vi "FF_AnkleTrajAdv.vi"(6 "Init":bool, 7 "dt":dbl=0.01 format="%0.2f", 8 "error in (no error)":errorcluster, 9 "AnkleVelocity":dbl[](array[numeric]), 10 "AnkleInGCS":dbl[](array[numeric]), 11 "Force Field Controller in":refnum<class "ForceField.lvclass">) -> (0 "error out":errorcluster, 1 "ClosestPoint":dbl[](array[numeric]), 2 "ForceXYZ":dbl[](array[numeric]), 3 "Force Field Controller out":refnum<class "ForceField.lvclass">, 4 "UpdateTrajPrev":bool, 5 "ForceNTD":dbl[](array[numeric]))   [LabVIEW 2016, in "ForceField.lvclass"]
uses:
  ForceField.lvclass
  ForceField.lvclass/ForceField.ctl
  <vilib>/ptbypt/NI_PtbyPt.lvlib
panel:
  out "ToeOffIdx":i32
  in  "3D":bool
  in  "Adv?":bool=TRUE
  out "weightPrev":dbl
  out "ClosePt 2":dbl[](array[numeric])
  in  "HalfWindow 2":i32=35
  in  "dXmin":dbl=0.2 format="%#_13g"
  in  "HalfWindow 1":i32=35
  out "ClosePt 1":dbl[](array[numeric])
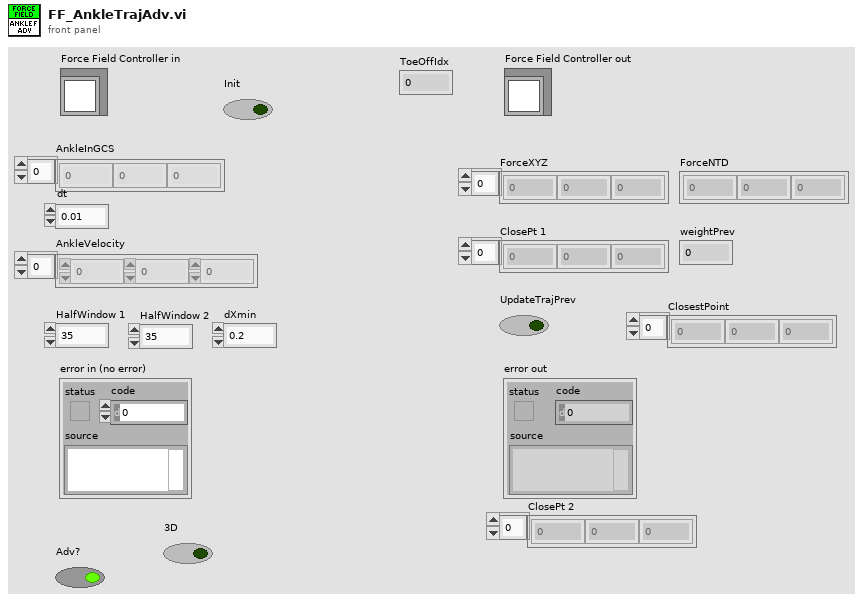
[diagram p1: front panel]
types:
  T1 = typedef "ForceField.lvclass/AnkleTrajPt.ctl" = cluster{"P1":dbl[], "P2":dbl[], "P1-P2":dbl[], "(P1-P2)^2":dbl}
  T2 = typedef "ForceField.lvclass/ForceNTD.ctl" = cluster{"Vn":dbl[], "Vt":dbl[], "Dmin":dbl}
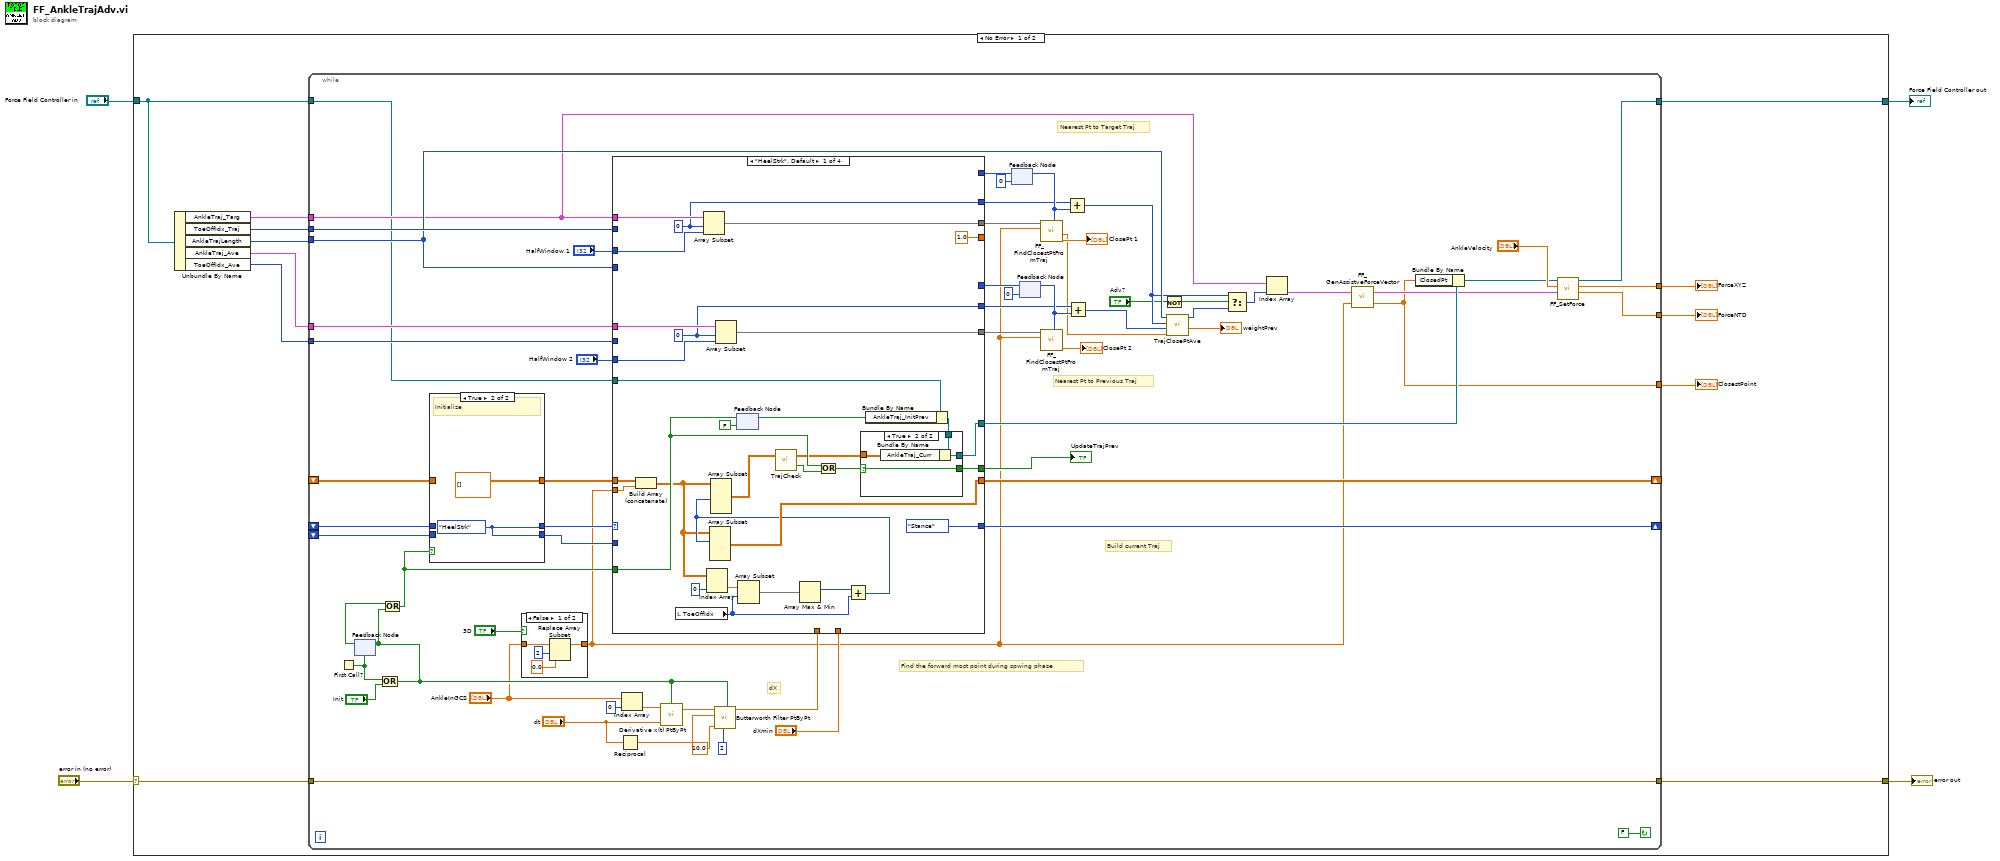
[diagram p0: block diagram]
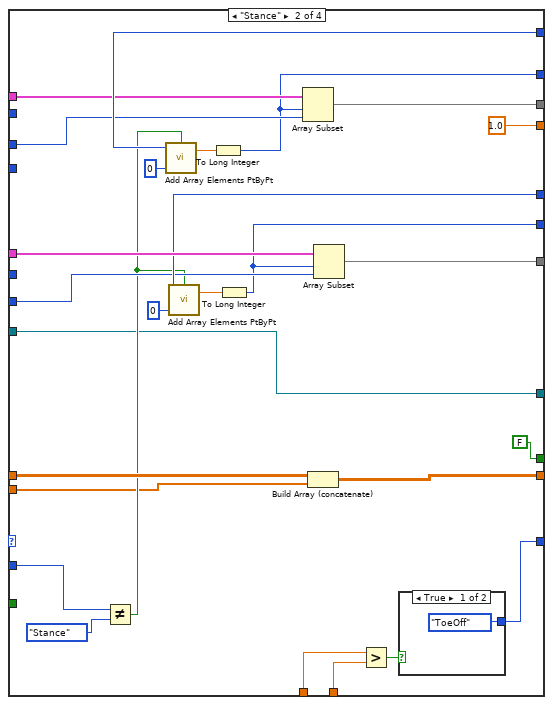
[diagram p4: hidden frame]
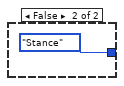
[diagram p5: hidden frame]
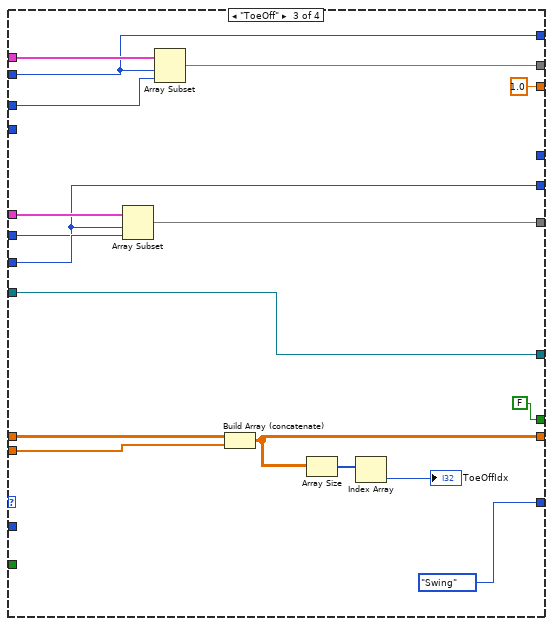
[diagram p6: hidden frame]
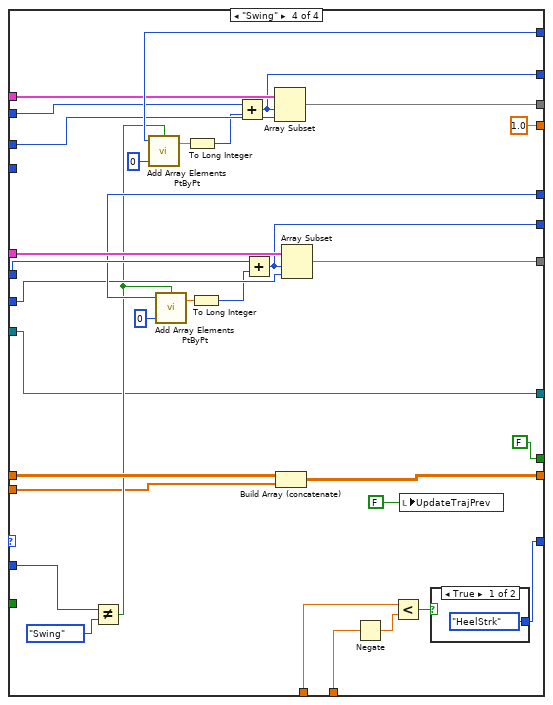
[diagram p7: hidden frame]
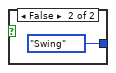
[diagram p8: hidden frame]
diagram:
  n1 = case shown="No Error" "error in (no error)" {
    selector: "error in (no error)" -> [w10 w211]
    tunnel: [w5 w211] -> w3
    tunnel: [w9 w210] -> w1
    tunnel: "Force Field Controller in" -> [w16 w210]
    frame No Error {
      n2 = Unbundle By Name(w16) -> ("AnkleTraj_Targ"=w15:T1[], "ToeOffIdx_Traj"=w14:i32, "AnkleTrajLength"=w13:i32, "AnkleTraj_Ave"=w12:T1[], "ToeOffIdx_Ave"=w11:i32)
      n3 = while {
        tunnel: w15 -> [w65]
        tunnel: w14 -> [w75]
        tunnel: w16 -> [w42]
        tunnel: [w21] -> w9
        shift-right: [w78] -> _
        shift-left: _ -> [w70]
        shift-left: _ -> [w68]
        shift-right: [w77] -> _
        shift-left: _ -> [w72]
        tunnel: w13 -> [w73]
        tunnel: w12 -> [w76]
        tunnel: w11 -> [w74]
        tunnel: w10 -> [w17]
        tunnel: [w20] -> w8
        tunnel: [w19] -> w7
        tunnel: [w18] -> w6
        tunnel: [w17] -> w5
        stop <- FALSE continue-if-true
        # "dX"
        # "Find the forward most point during spwing phase"
        # "Nearest Pt to Previous Traj"
        # "Build current Traj"
        # "Nearest Pt to Target Traj"
        n4 = First Call?() -> (First Call?: T/F=w28:bool)
        n5 = feedback #1(w28) -> (w66:bool)
        n6 = Or(x=w28, y="Init") -> (x .or. y?=w38:bool)
        n7 = feedback-in #1(w38) -> ()
        n8 = Or(x=w66, y=w38) -> (x .or. y?=w63:bool)
        n9 = case shown="True" w63 {
          tunnel: w72 -> [w207 _]
          tunnel: [w207 dbl[][] []] -> w71
          tunnel: w70 -> [w206 _]
          tunnel: [w206 w208] -> w69
          tunnel: w68 -> [w205 _]
          tunnel: [w205 w208] -> w67
          frame False {
          }
          frame True {
            w208 = enum16{"HeelStrk", "Stance", "ToeOff", "Swing"}."HeelStrk"
            # "Initialize"
          }
        }
        n10 = case shown="False" "3D" {
          tunnel: "AnkleInGCS" -> [w85 w86]
          tunnel: [w84 w86] -> w25
          frame False {
            n11 = Replace Array Subset(array=w85, new element=0.0 ("new element/subarray"), index=2) -> (w84:dbl[])
          }
          frame True {
          }
        }
        n12 = Reciprocal(x="dt") -> (1/x=w36:dbl)
        n13 = Index Array(array="AnkleInGCS", index=0) -> (element=w30:dbl)
        n14 = call <vilib>:"Derivative x(t) PtByPt.vi"("initialize"=w38, "dt"="dt", "x"=w30) -> ("dx/dt"=w40:dbl)  [unwired: 1 in, 1 out]
        n15 = call <vilib>:"Butterworth Filter PtByPt.vi"("initialize"=w38, "order"=2, "low cutoff freq: fl"=10.0, "sampling freq: fs"=w36, "x"=w40) -> ("Filtered x"=w31:dbl)  [unwired: 4 in, 1 out]
        n16 = feedback #2(0 ("IndexOfClosePt")) -> (w61:i32)
        n17 = feedback #3(0 ("IndexOfClosePt")) -> (w55:i32)
        n18 = case shown="\"HeelStrk\", Default" w69 {
          tunnel: w65 -> [w114 w142 w164 w188]
          tunnel: "HalfWindow 1" -> [w115 w149 w167 w201]
          tunnel: [w117 w146 w169 w198] -> w59
          tunnel: [enum16{"HeelStrk", "Stance", "ToeOff", "Swing"}."Stance" w145 enum16{"HeelStrk", "Stance", "ToeOff", "Swing"}."Swing" w196] -> w78
          tunnel: w61 -> [_ w150 _ w202]
          tunnel: w31 -> [_ w144 _ w195]
          tunnel: w67 -> [_ w141 _ w194]
          tunnel: [1.0 1.0 1.0 1.0] -> _
          tunnel: "dXmin" -> [_ w139 _ w191]
          tunnel: w25 -> [w104 w125 w157 w171]
          tunnel: [w100 w138 w155 w189] -> w77
          tunnel: w71 -> [w101 w137 w165 w190]
          tunnel: w73 -> [_ _ _ _]
          tunnel: w76 -> [w112 w135 w163 w183]
          tunnel: "HalfWindow 2" -> [w111 w132 w161 w180]
          tunnel: [w110 w133 w162 w179] -> w54
          tunnel: w75 -> [_ _ w160 w186]
          tunnel: w55 -> [_ w134 _ w181]
          tunnel: w74 -> [_ _ w159 w182]
          tunnel: [w108 w127 w159 w177] -> w51
          tunnel: [w109 w128 w160 w176] -> w49
          tunnel: w63 -> [w102 _ _ _]
          tunnel: w42 -> [w106 w126 w158 w172]
          tunnel: [w91 w126 w158 w172] -> w41
          tunnel: [w88 FALSE FALSE FALSE] -> w32
          frame "HeelStrk", Default {
            w108 = 0 ("index")
            w109 = 0 ("index")
            n19 = Build Array (concatenate)(w101, w104) -> (w98:dbl[][])
            n20 = local read "ToeOffIdx"() -> (w94:i32)
            n21 = Array Subset(array=w114, index=w109, length=w115) -> (w117:T1[])
            n22 = Index Array(array=w98, index (col)=0 ("disabled index (col)")) -> (element=w96:dbl[])  [unwired: 1 in]
            n23 = Array Subset(array=w112, index=w108, length=w111) -> (w110:T1[])
            n24 = feedback-in #4(w102) -> ()
            n25 = feedback #4(FALSE) -> (w105:bool)
            n26 = Array Subset(array=w96, index=w94) -> (w95:dbl[])  [unwired: 1 in]
            n27 = Array Max & Min(array=w95) -> (max index (indices)=w93:i32)  [unwired: 3 out]
            n28 = Add(x=w93, y=w94) -> (x+y=w99:i32)
            n29 = Array Subset(array=w98, index (row)=w99) -> (w100:dbl[][])  [unwired: 3 in]
            n30 = Array Subset(array=w98, length (row)=w99) -> (w89:dbl[][])  [unwired: 3 in]
            n31 = call "TrajCheck.vi"("Traj In"=w89) -> ("Good Trajectory?"=w103:bool, "Traj dup"=w87:dbl[][])  [unwired: 1 in]
            n32 = Or(x=w102, y=w103) -> (x .or. y?=w90:bool)
            n33 = Bundle By Name(cluster=w106, "AnkleTraj_InitPrev"=w105) -> (w92:refnum<class "ForceField.lvclass">)
            n34 = case shown="True" w90 {
              selector: w90 -> [w119 w121]
              tunnel: w92 -> [w118 w123]
              tunnel: [w118 w122] -> w91
              tunnel: [w119 w121] -> w88
              tunnel: w87 -> [_ w120]
              frame False {
              }
              frame True {
                n35 = Bundle By Name(cluster=w123, "AnkleTraj_Curr"=w120) -> (w122:refnum<class "ForceField.lvclass">)
              }
            }
          }
          frame "Stance" {
            n36 = Not Equal?(x=w141, y=enum16{"HeelStrk", "Stance", "ToeOff", "Swing"}."Stance") -> (x != y?=w131:bool)
            n37 = call <vilib>:"Add Array Elements PtByPt.vi"("initialize"=w131, "sample length"=0, "input data point"=w150) -> ("sum"=w130:dbl)  [unwired: 1 in, 1 out]
            n38 = call <vilib>:"Add Array Elements PtByPt.vi"("initialize"=w131, "sample length"=0, "input data point"=w134) -> ("sum"=w129:dbl)  [unwired: 1 in, 1 out]
            n39 = To Long Integer(number=w130) -> (32bit integer=w128:i32)
            n40 = To Long Integer(number=w129) -> (32bit integer=w127:i32)
            n41 = Array Subset(array=w142, index=w128, length=w149) -> (w146:T1[])
            n42 = Build Array (concatenate)(w137, w125) -> (w138:dbl[][])
            n43 = Array Subset(array=w135, index=w127, length=w132) -> (w133:T1[])
            n44 = Greater?(x=w144, y=w139) -> (0:w143:bool)
            n45 = case shown="True" w143 {
              tunnel: [enum16{"HeelStrk", "Stance", "ToeOff", "Swing"}."ToeOff" enum16{"HeelStrk", "Stance", "ToeOff", "Swing"}."Stance"] -> w145
              frame True {
              }
              frame False {
              }
            }
          }
          frame "ToeOff" {
            n46 = Array Subset(array=w163, index=w159, length=w161) -> (w162:T1[])
            n47 = Array Subset(array=w164, index=w160, length=w167) -> (w169:T1[])
            n48 = Build Array (concatenate)(w165, w157) -> (w155:dbl[][])
            n49 = Array Size(array=w155) -> (size(s)=w154:i32[])
            n50 = Index Array(array=w154) -> (element=→"ToeOffIdx":i32)  [unwired: 1 in]
          }
          frame "Swing" {
            n51 = Not Equal?(x=w194, y=enum16{"HeelStrk", "Stance", "ToeOff", "Swing"}."Swing") -> (x != y?=w178:bool)
            n52 = call <vilib>:"Add Array Elements PtByPt.vi"("initialize"=w178, "sample length"=0, "input data point"=w202) -> ("sum"=w187:dbl)  [unwired: 1 in, 1 out]
            n53 = call <vilib>:"Add Array Elements PtByPt.vi"("initialize"=w178, "sample length"=0, "input data point"=w181) -> ("sum"=w185:dbl)  [unwired: 1 in, 1 out]
            n54 = To Long Integer(number=w187) -> (32bit integer=w175:i32)
            n55 = To Long Integer(number=w185) -> (32bit integer=w174:i32)
            n56 = Add(x=w186, y=w175) -> (x+y=w176:i32)
            n57 = Add(x=w182, y=w174) -> (x+y=w177:i32)
            n58 = Array Subset(array=w188, index=w176, length=w201) -> (w198:T1[])
            n59 = Build Array (concatenate)(w190, w171) -> (w189:dbl[][])
            n60 = Array Subset(array=w183, index=w177, length=w180) -> (w179:T1[])
            n61 = Negate(x=w191) -> (-x=w192:dbl)
            n62 = Less?(x=w195, y=w192) -> (x < y?=w197:bool)
            n63 = local write "UpdateTrajPrev"(FALSE ("UpdateTrajPrev")) -> ()
            n64 = case shown="True" w197 {
              tunnel: [enum16{"HeelStrk", "Stance", "ToeOff", "Swing"}."HeelStrk" enum16{"HeelStrk", "Stance", "ToeOff", "Swing"}."Swing"] -> w196
              frame True {
              }
              frame False {
              }
            }
          }
        }
        "UpdateTrajPrev" <- w32
        n65 = call "FF_FindClosestPtFromTraj.vi"("AnkleInGCS"=w25, "AnkleTraj"=w59) -> ("ClosestPt"=→"ClosePt 1":dbl[], "DistanceToClosestPt"=w29:dbl, "IndexOfClosePt"=w50:i32)  [unwired: 5 in, 2 out]
        n66 = feedback-in #2(w50) -> ()
        n67 = call "FF_FindClosestPtFromTraj.vi"("AnkleInGCS"=w25, "AnkleTraj"=w54) -> ("ClosestPt"=→"ClosePt 2":dbl[], "IndexOfClosePt"=w52:i32)  [unwired: 5 in, 3 out]
        n68 = feedback-in #3(w52) -> ()
        n69 = Add(x=w49, y=w50) -> (x+y=w45:i32)
        n70 = Add(x=w51, y=w52) -> (x+y=w48:i32)
        n71 = Not(x="Adv?") -> (.not. x?=w43:bool)
        n72 = call "TrajClosePtAve.vi"("Dmin_Ave"=w29, "ClosePtIdx_Ave"=w48, "Dmin_Target"=w45, "ClosePtIdx_Target"=w73) -> ("weightTarget"=→"weightPrev":dbl, "ClosePtIdx_Ave"=w46:i32)  [unwired: 6 in]
        n73 = Select(t=w45, s=w43, f=w46) -> (s? t:f=w62:i32)
        n74 = Index Array(array=w65, index=w62) -> (element=w26:T1)
        n75 = call "FF_GenAssistveForceVector.vi"("AnkleInGCS"=w25, "Cloest Point on Traj"=w26) -> ("Closest Point in GCS"=w20:dbl[], "Assist Force NTD"=w24:T2)
        n76 = Bundle By Name(cluster=w41, "ClosedPt"=w20) -> (w22:refnum<class "ForceField.lvclass">)
        n77 = call "FF_SetForce.vi"("Assistive Force Vector"=w24, "AnkleVelocity"="AnkleVelocity", "Force Field Controller in"=w22) -> ("ForceNTD"=w18:dbl[], "ForceXYZ"=w19:dbl[], "Force Field Controller out"=w21:refnum<class "ForceField.lvclass">)  [unwired: 5 in, 1 out]
      }
      "ClosestPoint" <- w8
      "ForceXYZ" <- w7
      "ForceNTD" <- w6
    }
    frame Error {
    }
  }
  "error out" <- w3
  "Force Field Controller out" <- w1
